vi "hidSPD Setup Controller.vi"(8 "error in (no error)":errorcluster, 10 "hidSPD Controller Setup report":T1 {"HV_bias" format="%#_6p, V"; "TSet" format="%#_6p, DegC"}, 11 "spdDevSession in":T2={"spdRef"=0, "connected"=FALSE, "spdName"="", "specification"={"diod case"=enum."default", "type"=enum."Unknown", "frequency"=enum."Unknown"}, "hidSPD.Controller"={"TSet"=0.0, "HV_bias"=0.0, "DDS_stb_code"=0}, "hidSPD.Sturtup Values"={"TSet"=0.0, "HV_bias"=0.0, "DDS_stb_code"=0}} {"hidSPD.Sturtup Values"."HV_bias" format="%#_6p, V"; "hidSPD.Sturtup Values"."TSet" format="%#_6p, DegC"; "hidSPD.Controller"."HV_bias" format="%#_6p, V"; "hidSPD.Controller"."TSet" format="%#_6p, DegC"}) -> (0 "error out":errorcluster, 3 "spdDevSession out":T2={"spdRef"=0, "connected"=FALSE, "spdName"="", "specification"={"diod case"=enum."default", "type"=enum."Unknown", "frequency"=enum."Unknown"}, "hidSPD.Controller"={"TSet"=0.0, "HV_bias"=0.0, "DDS_stb_code"=0}, "hidSPD.Sturtup Values"={"TSet"=0.0, "HV_bias"=0.0, "DDS_stb_code"=0}} {"hidSPD.Sturtup Values"."HV_bias" format="%#_6p, V"; "hidSPD.Sturtup Values"."TSet" format="%#_6p, DegC"; "hidSPD.Controller"."HV_bias" format="%#_6p, V"; "hidSPD.Controller"."TSet" format="%#_6p, DegC"})   [LabVIEW 2018, in "hidSPDLibForLabView.lvlib"]
uses:
  hidSPDLibForLabView.lvlib
  hidSPD Controls/hidSPD Device Session.ctl
  hidSPD Controls/hidSPD.SPD specification.ctl
  hidSPD Controls/hidSPD SPD Diod Case.ctl
  hidSPD Controls/hidSPD SPD Type.ctl
  hidSPD Controls/hidSPD.STB Frequency.ctl
  hidSPD Controls/hidSPD Controller.ctl
  hidSPD Controls/hidSPD Controller Setup Report.ctl
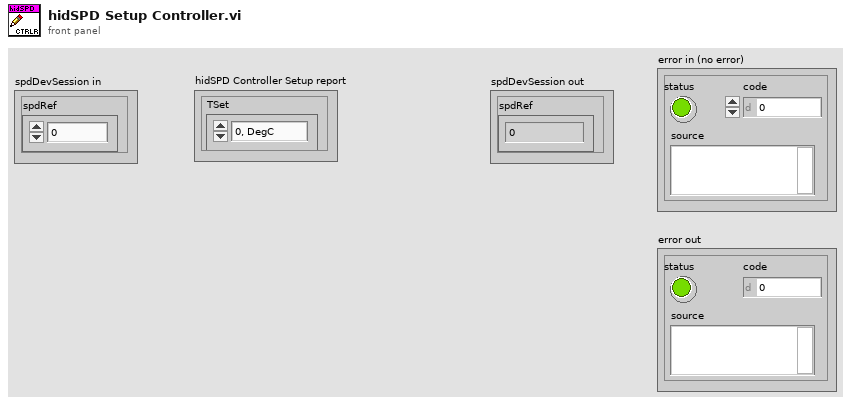
[diagram p1: front panel]
types:
  T1 = typedef "hidSPDLibForLabView.lvlib/hidSPD Controller Setup Report.ctl" = cluster{"TSet":sgl, "HV_bias":sgl, "DDS_stb_code":u16, "SPD_reset":u16, "MCU_reset":u16}
  T2 = typedef "hidSPDLibForLabView.lvlib/hidSPD Device Session.ctl" = cluster{"spdRef":u64, "connected":bool, "spdName":string, "specification":T3, "hidSPD.Controller":T7, "hidSPD.Sturtup Values":T7}
  T3 = typedef "hidSPDLibForLabView.lvlib/hidSPD.SPD specification.ctl" = cluster{"diod case":T4, "type":T5, "frequency":T6}
  T4 = typedef "hidSPDLibForLabView.lvlib/hidSPD SPD Diod Case.ctl" = enum16{"Unknown", "default", "butterfly"}
  T5 = typedef "hidSPDLibForLabView.lvlib/hidSPD SPD Type.ctl" = enum16{"Unknown", "Free Run", "Gate"}
  T6 = typedef "hidSPDLibForLabView.lvlib/hidSPD.STB Frequency.ctl" = enum16{"Unknown", "312", "1250"}
  T7 = typedef "hidSPDLibForLabView.lvlib/hidSPD Controller.ctl" = cluster{"TSet":sgl, "HV_bias":sgl, "DDS_stb_code":u16}
  T8 = enum16{"big-endian, network order", "native, host order", "little-endian"}
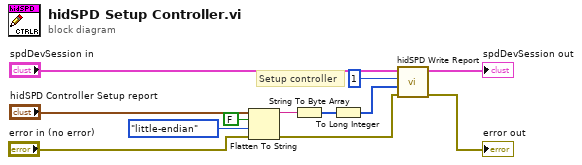
[diagram p0: block diagram]
diagram:
  # "Setup controller"
  n1 = Flatten To String(anything="hidSPD Controller Setup report", prepend array or string size? (T)=FALSE, byte order (0:big-endian, network order)=T8."little-endian", error in (no error)="error in (no error)") -> (data string=w9:string, error out=w6:errorcluster)  [unwired: 1 out]
  n2 = String To Byte Array(string=w9) -> (unsigned byte array=w8:u8[])
  n3 = To Long Integer(number=w8) -> (32bit integer=w7:i32[])
  n4 = call "hidSPD Write Report.vi"("error in (no error)"=w6, "data"=w7, "cmd"=1, "spdDevSession in"="spdDevSession in") -> ("error out"=→"error out":errorcluster, "spdDevSession out"=→"spdDevSession out":T2)  [unwired: 6 in]
